vi "getPathFromRRTTeam.vi"(8 "error in (no error)":errorcluster, 11 "Game in":refnum<class "Game.lvclass">) -> (0 "error out":errorcluster, 2 "RoboRef":refnum<class "Robot.lvclass">[](array[class]), 3 "Game out":refnum<class "Game.lvclass">)   [LabVIEW 2020, in "Game.lvclass"]
uses:
  Game.lvclass
  Robot_class/Robot.lvclass
  Game.lvclass/Game.ctl
  Team_class/Team.lvclass/Team.ctl
  Robot_class/Robot.lvclass/Robot.ctl
  Robot_class/Read id.vi
  Read Utilities.lvclass.vi
  Read OffensiveTeam.vi
  Read RRTTeam.vi
  Team_class/Read RobotRef.vi
  Ally_class/Ally.lvclass
  C:/RoboIME/SSL_AI/Team_class/Team.lvclass
  Utilities_class/Utilities.lvclass
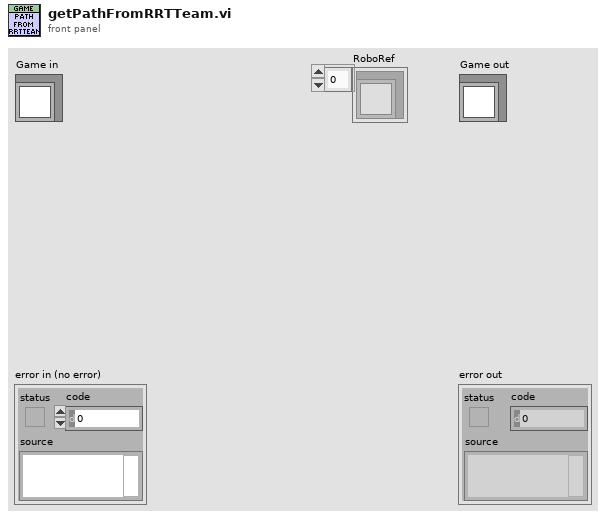
[diagram p1: front panel]
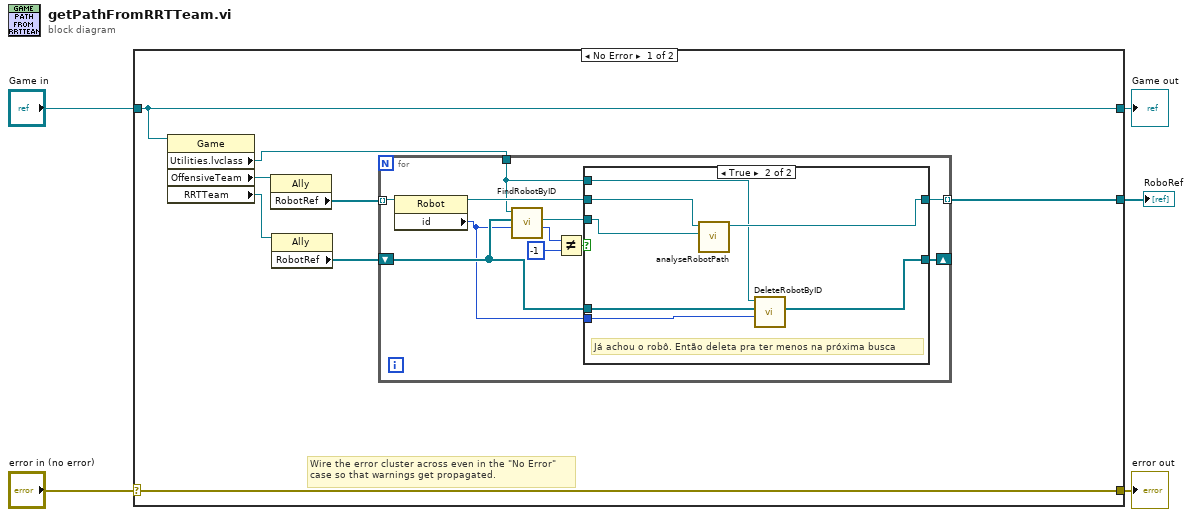
[diagram p0: block diagram]
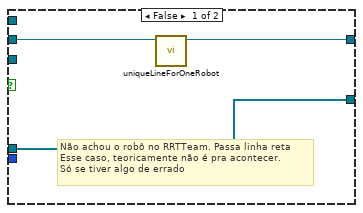
[diagram p2: hidden frame]
diagram:
  n1 = case shown="No Error" "error in (no error)" {
    selector: "error in (no error)" -> [w13 w36]
    tunnel: [w13 w36] -> w4
    tunnel: [w12 w35] -> w2
    tunnel: "Game in" -> [w12 w35]
    tunnel: [w6 _] -> w1
    frame No Error {
      # "Wire the error cluster across even in the \"No Error\"\ncase so that warnings get propagated."
      n2 = property class="Game"(reference=w12) -> ("Utilities.lvclass"=w7:refnum<class "Utilities.lvclass">, "OffensiveTeam"=w11:refnum<class "Ally.lvclass">, "RRTTeam"=w10:refnum<class "Ally.lvclass">)  [unwired: 1 in, 2 out]
      n3 = property class="Ally"(reference=w11) -> ("RobotRef"=w9:refnum<class "Robot.lvclass">[])  [unwired: 1 in, 2 out]
      n4 = property class="Ally"(reference=w10) -> ("RobotRef"=w8:refnum<class "Robot.lvclass">[])  [unwired: 1 in, 2 out]
      n5 = for {
        tunnel: w9 -> [w24] mode=indexing
        shift-right: [w16] -> _
        shift-left: w8 -> [w17]
        tunnel: w7 -> [w15]
        tunnel: [w19] -> w6 mode=indexing
        n6 = property class="Robot"(reference=w24) -> (reference out=w20:refnum<class "Robot.lvclass">, "id"=w14:i32)  [unwired: 1 in, 1 out]
        n7 = call "FindRobotByID.vi"("id"=w14, "RobotRef"=w17, "Utilities in"=w15) -> ("index"=w23:i32, "Robot"=w18:refnum<class "Robot.lvclass">)  [unwired: 5 in, 2 out]
        n8 = Not Equal?(x=w23, y=-1) -> (x != y?=w21:bool)
        n9 = case shown="True" w21 {
          tunnel: w20 -> [w26 w34]
          tunnel: [w25 w33] -> w19
          tunnel: w18 -> [_ w32]
          tunnel: w17 -> [w27 w31]
          tunnel: [w27 w30] -> w16
          tunnel: w15 -> [_ w29]
          tunnel: w14 -> [_ w28]
          frame False {
            # "Não achou o robô no RRTTeam. Passa linha reta\nEsse caso, teoricamente não é pra acontecer.\nSó se tiver algo de errado"
            n10 = call "uniqueLineForOneRobot.vi"("Robot in"=w26) -> ("Robot out"=w25:refnum<class "Robot.lvclass">)  [unwired: 10 in]
          }
          frame True {
            # "Já achou o robô. Então deleta pra ter menos na próxima busca"
            n11 = call "analyseRobotPath.vi"("RRTRobot in"=w32, "OffensiveRobot in"=w34) -> ("Robot out"=w33:refnum<class "Robot.lvclass">)  [unwired: 9 in]
            n12 = call-dynamic "DeleteRobotByID.vi"("id"=w28, "RobotRef"=w31, "Utilities in"=w29) -> ("RobotRef out"=w30:refnum<class "Robot.lvclass">[])  [unwired: 6 in, 2 out]
          }
        }
      }
    }
    frame Error {
    }
  }
  "error out" <- w4
  "Game out" <- w2
  "RoboRef" <- w1
